vi "Example_RateCounter.vi"() -> ()   [LabVIEW 2013]
panel:
  out "errorOut 2":errorcluster
  in  "Threshold Voltage":dbl min=-2.0 max=4.0 step=0.1 format="%#.3f"
  in  "Rate Measurement \nTime (us)":i32=1000000
  in  "nSlot":i32=5
  in  "nChassis":i32=1
  in  "partNumber":string="SD-PXE-TDC-H0002"
  out "countRate":i32
  in  "stop":bool
  in  "nChannel":i32
  out "errorOut":errorcluster
  # "Module Under Test"
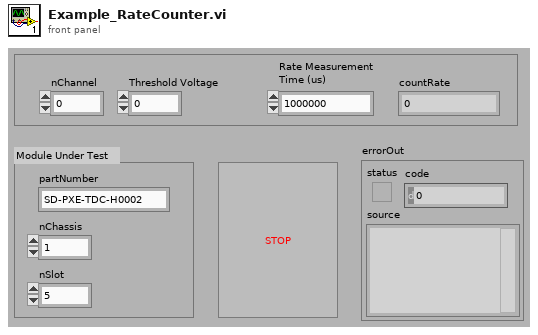
[diagram p1: front panel]
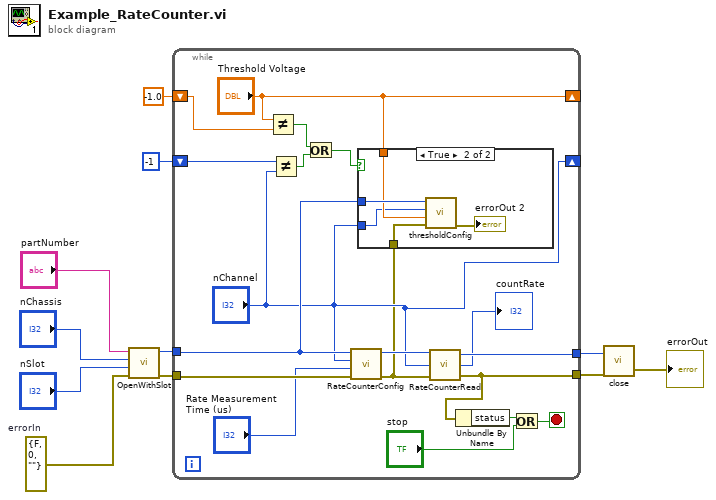
[diagram p0: block diagram]
diagram:
  w11 = errorcluster {"status"=FALSE, "code"=0, "source"=""}  # errorIn
  n1 = call <vilib>:"OpenWithSlot.vi"("errorIn"=w11, "nSlot"="nSlot", "nChassis"="nChassis", "partNumber"="partNumber") -> ("errorOut"=w7:errorcluster, "moduleID"=w6:i32)  [unwired: 2 in]
  n2 = while {
    tunnel: w7 -> [w27]
    tunnel: [w13] -> w5
    tunnel: w6 -> [w23]
    tunnel: [w29] -> w4
    shift-right: ["nChannel"] -> _
    shift-left: -1 ("nChannel") -> [w24]
    shift-right: ["Threshold Voltage"] -> _
    shift-left: -1.0 ("Threshold Voltage") -> [w22]
    stop <- w16 stop-if-true
    n3 = Not Equal?(x="Threshold Voltage", y=w22) -> (x != y?=w20:bool)
    n4 = Not Equal?(x=w24, y="nChannel") -> (x != y?=w21:bool)
    n5 = Or(x=w20, y=w21) -> (x .or. y?=w19:bool)
    n6 = call <vilib>:"RateCounterConfig.vi"("errorIn"=w27, "timeWindow"="Rate Measurement \nTime (us)", "nChannel"="nChannel", "moduleID"=w23) -> ("errorOut"=w12:errorcluster, "moduleIDout"=w26:i32)  [unwired: 2 in]
    n7 = case shown="True" w19 {
      tunnel: w23 -> [_ w34]
      tunnel: "nChannel" -> [_ w32]
      tunnel: "Threshold Voltage" -> [_ w33]
      tunnel: w12 -> [_ w31]
      frame False {
      }
      frame True {
        n8 = call <vilib>:"thresholdConfig.vi"("errorIn"=w31, "threshold"=w33, "nChannel"=w32, "moduleID"=w34) -> ("errorOut"=→"errorOut 2":errorcluster)  [unwired: 2 in, 1 out]
      }
    }
    n9 = call <vilib>:"RateCounterRead.vi"("errorIn"=w12, "nChannel"="nChannel", "moduleID"=w26) -> ("errorOut"=w13:errorcluster, "countRate"=→"countRate":i32, "moduleIDout"=w29:i32)
    n10 = Unbundle By Name(w13) -> ("status"=w15:bool)
    n11 = Or(x=w15, y="stop") -> (x .or. y?=w16:bool)
  }
  n12 = call <vilib>:"close.vi"("errorIn"=w5, "moduleID"=w4) -> ("errorOut"=→"errorOut":errorcluster)  [unwired: 1 in]
